vi "Read Protocol Type.vi"(8 "error in (no error)":errorcluster, 11 "Protocol Interface in":refnum<class "Protocol Interface.lvclass">) -> (0 "error out":errorcluster, 2 "Protocol Type":T1, 3 "Protocol Interface out":refnum<class "Protocol Interface.lvclass">)   [LabVIEW 2018, in "Protocol Interface.lvlib" / "Protocol Interface.lvclass"]
uses:
  Protocol Interface.lvclass
  Ctls/Protocol Type.ctl
  Protocol Interface.lvclass/Protocol Interface.ctl
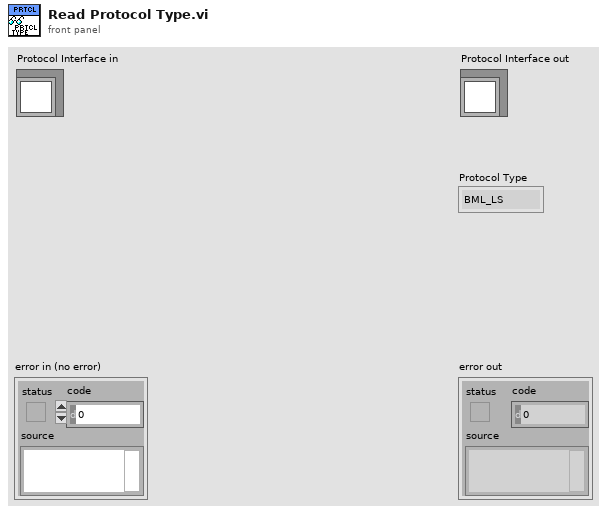
[diagram p1: front panel]
types:
  T1 = typedef "Protocol Type.ctl" = enum16{"BML_LS", "BML_HS", "SPI_3W", "SPI_4W"}
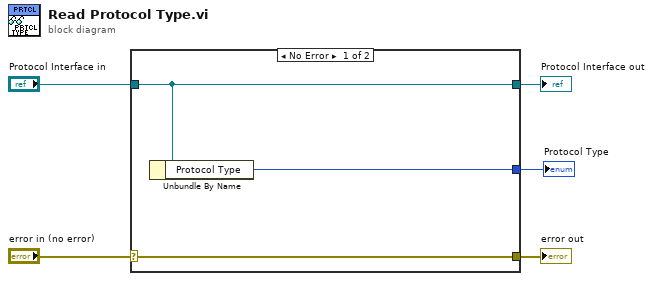
[diagram p0: block diagram]
diagram:
  n1 = case shown="No Error" "error in (no error)" {
    selector: "error in (no error)" -> [w8 w9]
    tunnel: [w8 w9] -> w4
    tunnel: [w7 w10] -> w2
    tunnel: "Protocol Interface in" -> [w7 w10]
    tunnel: [w6 _] -> w1
    frame No Error {
      n2 = Unbundle By Name(w7) -> ("Protocol Type"=w6:T1)
    }
    frame Error {
    }
  }
  "error out" <- w4
  "Protocol Interface out" <- w2
  "Protocol Type" <- w1
